vi "Init Group.vi"(8 "error in (no error)":errorcluster, 11 "Group in":refnum<class "Group.lvclass">) -> (0 "error out":errorcluster, 3 "Group out":refnum<class "Group.lvclass">)   [LabVIEW 2020, in "Vecto.lvlib" / "Group.lvclass"]
uses:
  Group.lvclass
  Group.lvclass/Group.ctl
  Ref.ctl
  GroupAbstract/GroupAbstract.lvclass
  Group Config/Group Config.lvclass
  C:/dev/lv20CE/relink/lv-vecto/Vecto/GroupAbstract/GroupAbstract.lvclass
  C:/dev/lv20CE/relink/lv-vecto/Vecto/Group/Group.lvclass
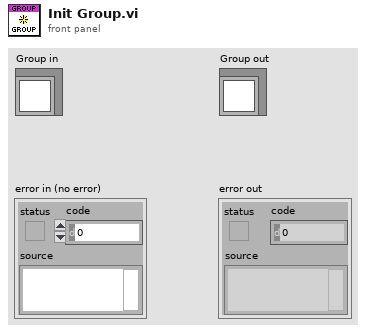
[diagram p1: front panel]
types:
  T1 = typedef "Vecto.lvlib/Group.lvclass/Ref.ctl" = cluster{"Scaled":dbl[], "Timestamp":dbl[], "Raw":dbl[]}
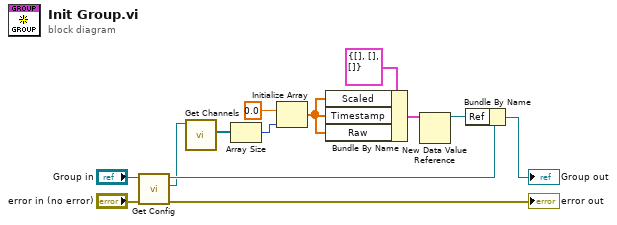
[diagram p0: block diagram]
diagram:
  n1 = call "Get Config.vi"("error in (no error)"="error in (no error)", "GroupAbstract in"="Group in") -> ("error out"=→"error out":errorcluster, "Config"=w2:refnum<class "Group Config.lvclass">, "GroupAbstract out"=w3:refnum<class "Group.lvclass">)  [unwired: 7 in]
  n2 = call "Get Channels.vi"("Group Config in"=w2) -> ("Channels"=w1:refnum<class "Channel Config.lvclass">[])  [unwired: 8 in, 2 out]
  n3 = Array Size(array=w1) -> (size(s)=w10:i32)
  n4 = Initialize Array(0.0 ("element"), w10) -> (w8:dbl[])
  n5 = Bundle By Name(cluster=T1 {"Scaled"=[], "Timestamp"=[], "Raw"=[]} ("Ref"), "Scaled"=w8, "Timestamp"=w8, "Raw"=w8) -> (w11:T1)
  n6 = New Data Value Reference(data value=w11) -> (data value reference=w6:refnum<data-value>)  [unwired: 1 in, 1 out]
  n7 = Bundle By Name(cluster=w3, "Ref"=w6) -> (→"Group out":refnum<class "Group.lvclass">)
